vi "Deadband and Scale.vi"(8 "Square Inputs":bool, 9 "Scaler (0-1)":dbl=1.0, 10 "Dead Zone (abs)":dbl=0.1, 11 "Input":dbl) -> (3 "Output":dbl)   [LabVIEW 2014]
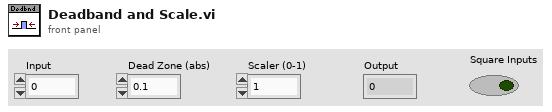
[diagram p1: front panel]
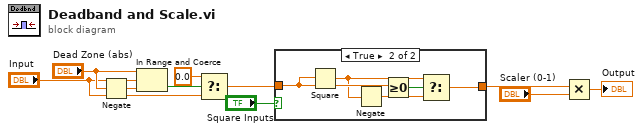
[diagram p0: block diagram]
diagram:
  n1 = Negate(x="Dead Zone (abs)") -> (-x=w9:dbl)
  n2 = In Range and Coerce(upper limit="Dead Zone (abs)", x="Input", lower limit=w9) -> (In Range?=w10:bool)  [unwired: 1 out]
  n3 = Select(t=0.0, s=w10, f="Input") -> (s? t:f=w2:dbl)
  n4 = case shown="True" "Square Inputs" {
    tunnel: [w11 w16] -> w1
    tunnel: w2 -> [w11 w15]
    frame False {
    }
    frame True {
      n5 = Square(x=w15) -> (x^2=w13:dbl)
      n6 = Negate(x=w13) -> (-x=w14:dbl)
      n7 = Greater Or Equal To 0?(x=w15) -> (x >= 0?=w12:bool)
      n8 = Select(t=w13, s=w12, f=w14) -> (s? t:f=w16:dbl)
    }
  }
  n9 = Multiply(x=w1, y="Scaler (0-1)") -> (x*y=→"Output":dbl)
